vi "Optoelectronic Data.vi"() -> (0 "Optoelectronic Data":T1)   [LabVIEW 2014]
uses:
  Optoelectronic Data.ctl
  Optoelectronic Refnums.ctl
  support/Instrument Status.ctl
  Plot Data/Optical Spectrum Plot Refnum.ctl
  Plot Data/Electrical Data Plot Refnums.ctl
  Optoelectronic Initialize.ctl
panel:
  # "LICENSED MATERIALS – PROPERTY OF IBM\nCopyright IBM Corp. 2016,\nALL RIGHTS RESERVED"
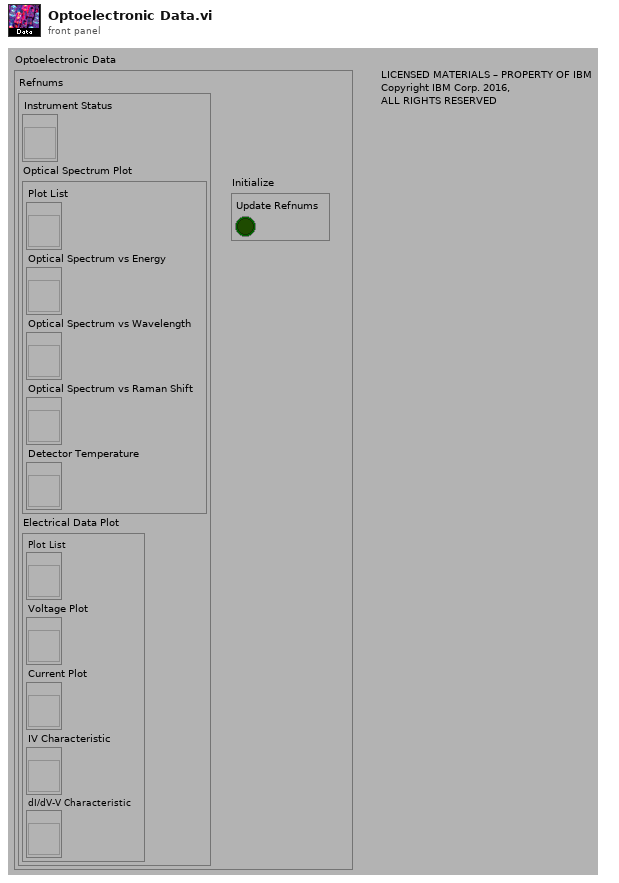
[diagram p1: front panel]
types:
  T1 = typedef "Optoelectronic Data.ctl" = cluster{"Refnums":T2, "Initialize":T5}
  T2 = typedef "Optoelectronic Refnums.ctl" = cluster{"Instrument Status":refnum<vi>, "Optical Spectrum Plot":T3, "Electrical Data Plot":T4}
  T3 = typedef "Optical Spectrum Plot Refnum.ctl" = cluster{"Plot List":refnum<vi>, "Optical Spectrum vs Energy":refnum<vi>, "Optical Spectrum vs Wavelength":refnum<vi>, "Optical Spectrum vs Raman Shift":refnum<vi>, "Detector Temperature":refnum<vi>}
  T4 = typedef "Electrical Data Plot Refnums.ctl" = cluster{"Plot List":refnum<vi>, "Voltage Plot":refnum<vi>, "Current Plot":refnum<vi>, "IV Characteristic":refnum<vi>, "dI/dV-V Characteristic":refnum<vi>}
  T5 = typedef "Optoelectronic Initialize.ctl" = cluster{"Update Refnums":bool}
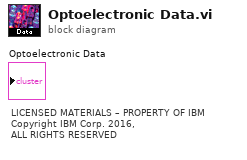
[diagram p0: block diagram]
diagram:
  # "LICENSED MATERIALS – PROPERTY OF IBM\nCopyright IBM Corp. 2016,\nALL RIGHTS RESERVED"
